vi "TPM with correction version 10-3-compare-1 scale factor_20180124.vi"() -> ()   [LabVIEW 2018]
uses:
  Casao LabVIEW SDK 1.0.5/Haso/Data Haso/Wavefront parameters.ctl
  Casao LabVIEW SDK 1.0.5/Casao/Casao/Loop prefs.ctl
  Casao LabVIEW SDK 1.0.5/Haso/Data Haso/DataHaso.ctl
  <vilib>/Utility/file.llb/Read From Spreadsheet File (DBL).vi
  <vilib>/Utility/file.llb/Write To Spreadsheet File (DBL).vi
panel:
  in  "Scale factor":dbl=1.0
  out "output path":path
  out "Model Coefficients (µm) after":sgl[](array[numeric])
  out "Model Coefficients (µm) before":sgl[](array[numeric])
  in  "stop":bool
  out "Slice now":dbl
  in  "Iteration #":u16(ring)=1 items=["1"=1, "2"=2, "3"=3, "4"=4, "5"=5]
  in  "AoExp Time":dbl(ring)=0.5 items=["0.2s"=0.2, "0.5s"=0.5, "1.0s"=1.0, "1.5s"=1.5]
  out "after correction":T1
  in  "Filter y tilt":bool=TRUE
  in  "Filter x tilt":bool=TRUE
  in  "Curvature filter":bool=TRUE
  out "PV":dbl
  out "RMS":dbl
  in  "Matrix path":path=path "F:/Min_Data/20180327_conf_calibration/CM32.aomc"
  in  "Offset path":path=path "F:/Min_Data/100nm bead correction.dat"
  out "Camera image":u32[][](graph)
  out "RMS":dbl
  out "PV":dbl
  out "before correction":T1
  in  "Curvature filter":bool=TRUE
  in  "Filter y tilt":bool=TRUE
  in  "Filter x tilt":bool=TRUE
  out "after correction":dbl[][](graph) caption="Wavefront"
  out "before correction":dbl[][](graph) caption="Wavefront"
  in  "ImExp Time (s)":dbl(ring)=0.5 items=["0.2"=0.2, "0.5"=0.5, "1.0"=1.0, "4.0"=4.0, "8.0"=8.0]
  in  "Step size(um)":dbl
  in  "Laser Power%(0-100)":dbl=50.0
  in  "Slices #":dbl=1.0
  in  "Average Frame #":dbl=10.0
  in  "Correction":bool
  # "OFF"
  # "ON"
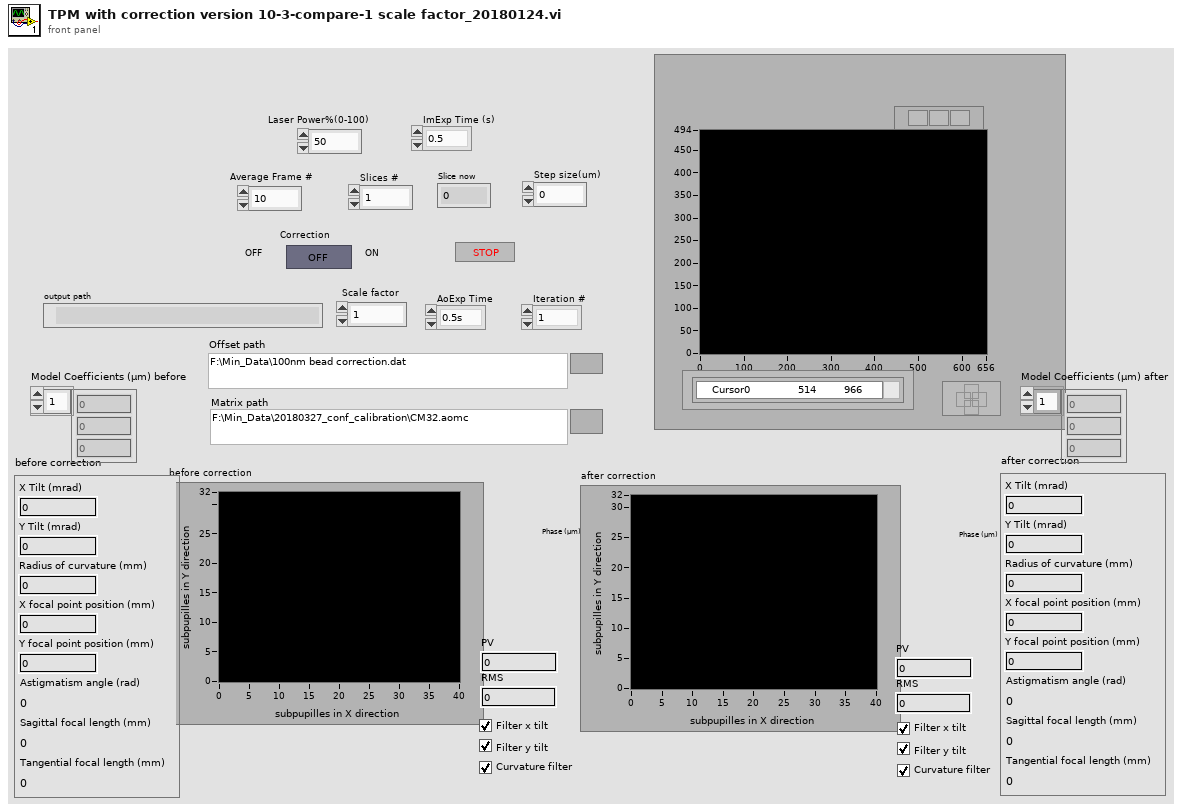
[diagram p1: front panel]
types:
  T1 = typedef "Wavefront parameters.ctl" = cluster{"X Tilt (mrad)":sgl, "Y Tilt (mrad)":sgl, "Radius of curvature (mm)":sgl, "X focal point position (mm)":sgl, "Y focal point position (mm)":sgl, "Astigmatism angle (rad)":sgl, "Sagittal focal length (mm)":sgl, "Tangential focal length (mm)":sgl}
  T2 = typedef "Loop prefs.ctl" = cluster{"Filter tilt on measurement (closed loop)":bool, "Correction gain (closed loop)":sgl, "Limit of subapertures off in CGP (%)":sgl, "Limit of saturated actuators (%)":sgl}
  T3 = cluster{"Filtre tilt X":bool, "Filtre tilt Y":bool, "Filtre courbure":bool}
  T4 = typedef "DataHaso.ctl" = i32
  T5 = cluster{"Measurement":T4, "Target":T4, "Manual target":T4}
  T6 = cluster{"Target for tilt":T4, "Target for focus":T4, "Target for all other aberrations":T4}
  T7 = typedef "Camera.ctl" = i32
  T8 = typedef "PhaseModul.ctl" = i32
  T9 = typedef "Haso.ctl" = i32
  T10 = typedef "Casao.ctl" = i32
  T11 = typedef "Image Compat.ctl" = cluster{"Signed/unsigned":bool, "Number of bits":T12, "Internal object id":i32, "Internal data id":i32}
  T12 = typedef "Data alignment enum.ctl" = enum16{"8", "16", "32"}
  T13 = typedef "Reconstruction prefs.ctl" = cluster{"Reconstruction type":enum16{"Modal", "Zonal"}, "Polynomial type":enum16{"Zernike", "Legendre"}, "Modal reconstruction prefs":T14, "Zonal reconstruction prefs":T17}
  T14 = typedef "Modal reconstruction prefs.ctl" = cluster{"Number of coefficients":u32, "Filtered coefficients":u32[], "RMS Zernike normalization":bool, "Matrix inversion method":u16, "Add zonal residual to modal fit ":bool, "Detection prefs":T15}
  T15 = typedef "PupilDetectionPrefs.ctl" = cluster{"Automatic pupil detection":bool, "Central occultation pupil":bool, "Semi-automatic pupil detection (find radius)":bool, "Semi-automatic pupil detection (find center)":bool, "Automatic pupil detection mode":enum16{"Contained", "Containing"}, "Start coordinates":cluster{"Pupil center (Zernike)":T16, "Pupil radius (Zernike)":sgl, "Pupil center (Legendre)":T16, "Pupil halfsize (Legendre)":T16}}
  T16 = typedef "Point2Df.ctl" = cluster{"X":sgl, "Y":sgl}
  T17 = typedef "Zonal reconstruction prefs.ctl" = cluster{"Number of weak iterations":u16, "Number of max iterations":u32, "Residual limit":sgl}
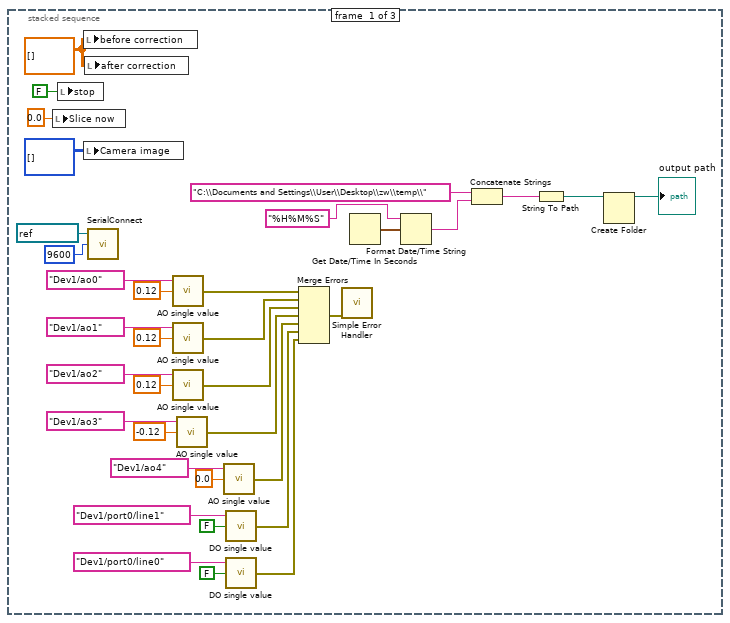
[diagram p2: hidden frame]
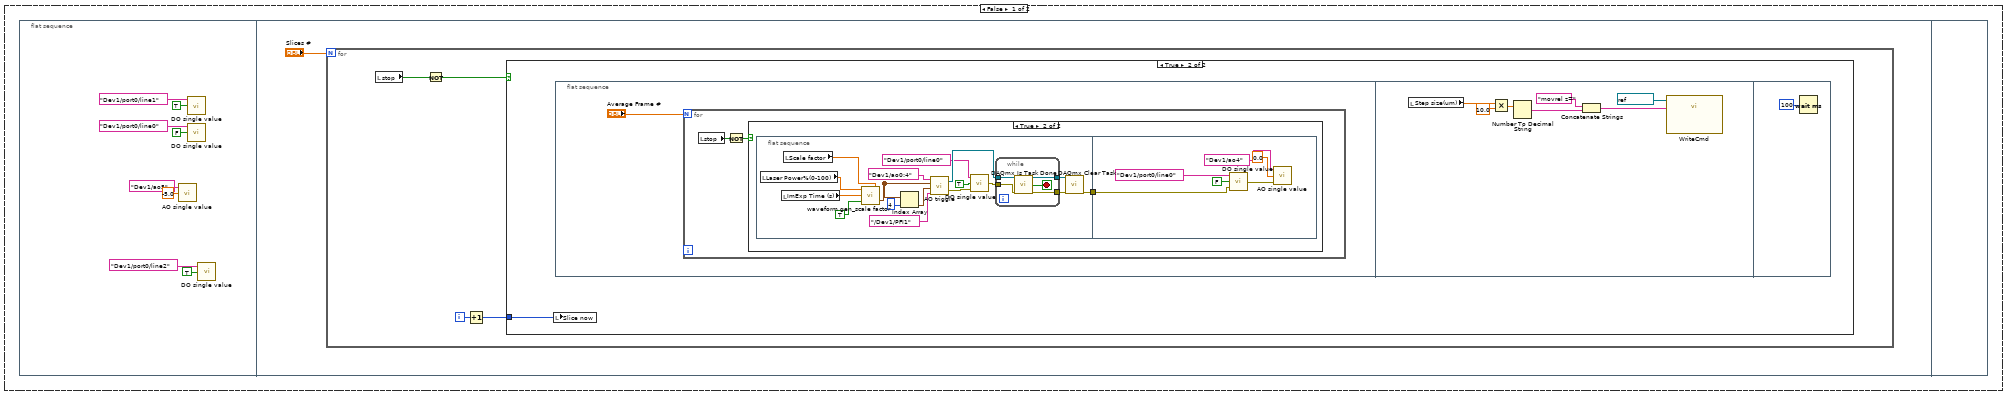
[diagram p3: hidden frame]
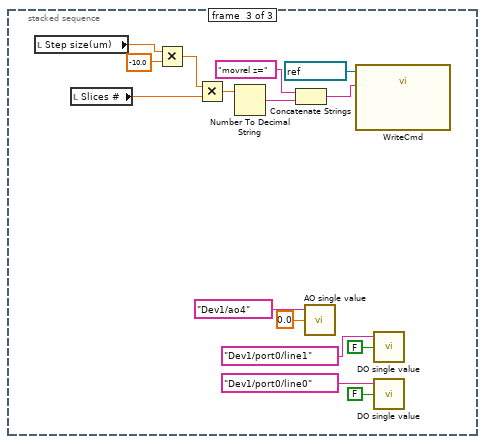
[diagram p11: hidden frame]
diagram:
  n1 = stacked-sequence {
    frame #0 {
      w34 = dbl[][] [] ("before correction")
      n2 = local write "Slice now"(0.0 ("Slice now")) -> ()
      n3 = local write "stop"(FALSE ("stop")) -> ()
      n4 = local write "before correction"(w34) -> ()
      n5 = local write "Camera image"(u32[][] [] ("Camera image")) -> ()
      n6 = local write "after correction"(w34) -> ()
      n7 = call "SerialConnect.vi"("baud rate (9600)"=u32 9600, "VISA resource name"=refnum<visa-resource-name> "COM1") -> ()  [unwired: 1 in, 3 out]
      n8 = call "AO single value.vi"("data"=0.12, "physical channels"=tag "Dev1/ao0") -> ("error out"=w17:errorcluster)  [unwired: 1 in]
      n9 = call "AO single value.vi"("data"=0.12, "physical channels"=tag "Dev1/ao1") -> ("error out"=w16:errorcluster)  [unwired: 1 in]
      n10 = call "AO single value.vi"("data"=0.12, "physical channels"=tag "Dev1/ao2") -> ("error out"=w15:errorcluster)  [unwired: 1 in]
      n11 = call "AO single value.vi"("data"=-0.12, "physical channels"=tag "Dev1/ao3") -> ("error out"=w14:errorcluster)  [unwired: 1 in]
      n12 = call "AO single value.vi"("data"=0.0, "physical channels"=tag "Dev1/ao4") -> ("error out"=w13:errorcluster)  [unwired: 1 in]
      n13 = call "DO single value.vi"("data"=FALSE, "lines"=tag "Dev1/port0/line1") -> ("error out"=w12:errorcluster)  [unwired: 1 in]
      n14 = call "DO single value.vi"("data"=FALSE, "lines"=tag "Dev1/port0/line0") -> ("error out"=w10:errorcluster)  [unwired: 1 in]
      n15 = Merge Errors(w17, w16, w15, w14, w13, w12, w10) -> (w11:errorcluster)
      n16 = call <vilib>:"Simple Error Handler.vi"("error in (no error)"=w11) -> ()  [unwired: 4 in, 5 out]
      n17 = Get Date/Time In Seconds() -> (seconds since 1Jan1904=w7:timestamp)
      n18 = Format Date/Time String(time format string (%c)="%H%M%S", seconds (now)=w7) -> (date/time string=w4:string)  [unwired: 1 in]
      n19 = Concatenate Strings("C:\\Documents and Settings\\User\\Desktop\\zw\\temp\\" ("string"), w4) -> (w3:string)
      n20 = String To Path(string=w3) -> (path=w2:path)
      n21 = Create Folder(path (use dialog)=w2) -> (created path=→"output path":path)  [unwired: 2 in, 2 out]
    }
    frame #1 {
      n22 = case shown="True" "Correction" {
        frame False {
          n23 = flat-sequence {
            frame #0 {
              n24 = call "AO single value.vi"("data"=-5.0, "physical channels"=tag "Dev1/ao5") -> ()  [unwired: 1 in, 1 out]
              n25 = call "DO single value.vi"("data"=TRUE, "lines"=tag "Dev1/port0/line1") -> ()  [unwired: 1 in, 1 out]
              n26 = call "DO single value.vi"("data"=FALSE, "lines"=tag "Dev1/port0/line0") -> ()  [unwired: 1 in, 1 out]
              n27 = call "DO single value.vi"("data"=TRUE, "lines"=tag "Dev1/port0/line2") -> ()  [unwired: 1 in, 1 out]
            }
            frame #1 {
              n28 = for {
                N: "Slices #" -> [_]
                i -> [w49]
                n29 = local read "stop"() -> (w47:bool)
                n30 = Not(x=w47) -> (.not. x?=w46:bool)
                n31 = Increment(x=w49) -> (x+1=w48:i32)
                n32 = case shown="True" w46 {
                  tunnel: w48 -> [_ w50]
                  frame False {
                  }
                  frame True {
                    n33 = local write "Slice now"(w50) -> ()
                    n34 = flat-sequence {
                      frame #0 {
                        n35 = for {
                          N: "Average Frame #" -> [_]
                          n36 = local read "stop"() -> (w52:bool)
                          n37 = Not(x=w52) -> (.not. x?=w53:bool)
                          n38 = case shown="True" w53 {
                            frame False {
                            }
                            frame True {
                              n39 = flat-sequence {
                                tunnel: [w60] -> w54
                                tunnel: w54 -> [w78]
                                frame #0 {
                                n40 = local read "Laser Power%(0-100)"() -> (w56:dbl)
                                n41 = local read "ImExp Time (s)"() -> (w57:dbl)
                                n42 = local read "Scale factor"() -> (w55:dbl)
                                n43 = call "waveform gen_scale factor.vi"("Scale factor"=w55, "Boolean"=TRUE, "Exposure Time (s)"=w57, "Laser Power%(0-100)"=w56) -> ("waveform"=w59:waveform(dbl)[])
                                n44 = Index Array(array=w59, index=4) -> (element=w68:waveform(dbl))
                                n45 = call "AO triggle.vi"("physical channels"=tag "Dev1/ao0:4", "data"=w59, "waveform"=w68, "trig source"=tag "/Dev1/PFI1") -> ("task out"=w65:refnum<k21>, "error out"=w62:errorcluster)  [unwired: 1 in]
                                n46 = call "DO single value.vi"("error in"=w62, "data"=TRUE, "lines"=tag "Dev1/port0/line0") -> ("error out"=w61:errorcluster)
                                n47 = while {
                                tunnel: [w76] -> w71
                                tunnel: [w75] -> w70
                                tunnel: w65 -> [w73]
                                tunnel: w61 -> [w72]
                                stop <- w74 stop-if-true
                                n48 = call <vilib>:"DAQmx Is Task Done.vi"("task/channels in"=w73, "error in"=w72) -> ("task out"=w76:refnum<k21>, "task done?"=w74:bool, "error out"=w75:errorcluster)  [unwired: 11 in]
                                }
                                n49 = call <vilib>:"DAQmx Clear Task.vi"("task in"=w71, "error in"=w70) -> ("error out"=w60:errorcluster)  [unwired: 13 in]
                                }
                                frame #1 {
                                n50 = call "DO single value.vi"("error in"=w78, "data"=FALSE, "lines"=tag "Dev1/port0/line0") -> ("error out"=w77:errorcluster)
                                n51 = call "AO single value.vi"("error in"=w77, "data"=0.0, "physical channels"=tag "Dev1/ao4") -> ()  [unwired: 1 out]
                                }
                              }
                            }
                          }
                        }
                      }
                      frame #1 {
                        n52 = local read "Step size(um)"() -> (w83:dbl)
                        n53 = Multiply(x=w83, y=10.0) -> (x*y=w85:dbl)
                        n54 = Number To Decimal String(number=w85) -> (decimal integer string=w88:string)  [unwired: 1 in]
                        n55 = Concatenate Strings("movrel z=", w88) -> (w87:string)
                        n56 = call "WriteCmd.vi"("Command"=w87, "VISA resource name"=refnum<visa-resource-name> "COM1") -> ()  [unwired: 1 in, 1 out]
                      }
                      frame #2 {
                        n57 = Wait (ms)(milliseconds to wait=u32 100) -> ()  [unwired: 1 out]
                      }
                    }
                  }
                }
              }
            }
            frame #2 {
            }
          }
        }
        frame True {
          n58 = flat-sequence {
            tunnel: [w106] -> w98
            tunnel: [w108] -> w97
            tunnel: [w107] -> w96
            tunnel: [w106] -> w95
            tunnel: [w105] -> w94
            tunnel: [w104] -> w92
            tunnel: [w99] -> w91
            tunnel: w98 -> [w125]
            tunnel: w97 -> [w124]
            tunnel: w96 -> [w123]
            tunnel: w95 -> [w119]
            tunnel: w94 -> [w117]
            tunnel: [w122] -> w93
            tunnel: w92 -> [w121]
            tunnel: w91 -> [w115]
            tunnel: w93 -> [w651]
            frame #0 {
              n59 = call "AO single value.vi"("data"=0.0, "physical channels"=tag "Dev1/ao4") -> ()  [unwired: 1 in, 1 out]
              n60 = local read "AoExp Time"() -> (w109:dbl)
              n61 = call-poly <vilib>:"Read From Spreadsheet File.vi"("format (%.3f)"="%.8f", "file path (dialog if empty)"="Offset path") -> ("first row"=w99:dbl[])  [unwired: 5 in, 4 out]
              n62 = call "DO single value.vi"("data"=TRUE, "lines"=tag "Dev1/port0/line1") -> ()  [unwired: 1 in, 1 out]
              n63 = call "DO single value.vi"("data"=FALSE, "lines"=tag "Dev1/port0/line0") -> ()  [unwired: 1 in, 1 out]
              n64 = call "AO init.vi"("Exposure duration specified (s)"=w109, "Commands in"=w99, "Matrix path"="Matrix path") -> ("error out"=w106:errorcluster, "Camera"=w108:T7, "Mirror"=w104:T8, "Haso"=w107:T9, "Casao"=w105:T10)  [unwired: 3 in, 1 out]
            }
            frame #1 {
              n65 = local read "Slices #"() -> (w126:dbl)
              n66 = call "Casao Set Preferences.vi"("error in (no error)"=w119, "Loop preferences"=T2 {"Filter tilt on measurement (closed loop)"=FALSE, "Correction gain (closed loop)"=0.75, "Limit of subapertures off in CGP (%)"=0.0, "Limit of saturated actuators (%)"=0.0}, "Casao"=w117) -> ("error out"=w118:errorcluster, "Casao (dup)"=w116:T10)  [unwired: 3 in]
              n67 = for {
                N: w126 -> [_]
                tunnel: w125 -> [w142]
                tunnel: w124 -> [w141]
                tunnel: w123 -> [w140]
                tunnel: w118 -> [w128]
                tunnel: [w139] -> w122
                tunnel: w121 -> [w130]
                tunnel: w116 -> [w138]
                tunnel: w115 -> [w131]
                i -> [w134]
                n68 = local read "stop"() -> (w136:bool)
                n69 = call "PhaseModul apply command.vi"("error in (no error)"=w128, "Commands in"=w131, "Mirror"=w130) -> ("error out"=w127:errorcluster, "Mirror (dup)"=w129:T8)  [unwired: 2 in, 1 out]
                n70 = Increment(x=w134) -> (x+1=w137:i32)
                n71 = local write "Slice now"(w137) -> ()
                n72 = Not(x=w136) -> (.not. x?=w135:bool)
                n73 = case shown="True" w135 {
                  tunnel: w142 -> [_ w177]
                  tunnel: w141 -> [_ w176]
                  tunnel: w140 -> [_ w175]
                  tunnel: w127 -> [_ w174]
                  tunnel: [w143 w171] -> w139
                  tunnel: w129 -> [_ w173]
                  tunnel: w138 -> [w143 w172]
                  frame False {
                  }
                  frame True {
                    n74 = flat-sequence {
                      tunnel: w172 -> [w182]
                      tunnel: w173 -> [w183]
                      tunnel: w174 -> [w184]
                      tunnel: w175 -> [w185]
                      tunnel: w176 -> [w186]
                      tunnel: w177 -> [w187]
                      tunnel: [w187] -> w149
                      tunnel: [w186] -> w148
                      tunnel: [w185] -> w147
                      tunnel: [w184] -> w146
                      tunnel: [w183] -> w145
                      tunnel: [w182] -> w144
                      tunnel: [w222] -> w170
                      tunnel: [w221] -> w169
                      tunnel: [w220] -> w168
                      tunnel: [w215] -> w167
                      tunnel: [w216] -> w166
                      tunnel: [w217] -> w165
                      tunnel: w149 -> [w222]
                      tunnel: w148 -> [w221]
                      tunnel: w147 -> [w220]
                      tunnel: w146 -> [w216]
                      tunnel: w145 -> [w217]
                      tunnel: w144 -> [w215]
                      tunnel: w170 -> [w264]
                      tunnel: w169 -> [w263]
                      tunnel: w168 -> [w262]
                      tunnel: w167 -> [w261]
                      tunnel: w166 -> [w260]
                      tunnel: [w240] -> w164
                      tunnel: [w239] -> w163
                      tunnel: [w235] -> w162
                      tunnel: [w233] -> w161
                      tunnel: [w231] -> w160
                      tunnel: w165 -> [w226]
                      tunnel: [w225] -> w159
                      tunnel: [w223] -> w158
                      tunnel: w164 -> [w406]
                      tunnel: w163 -> [w405]
                      tunnel: w162 -> [w403]
                      tunnel: w161 -> [w402]
                      tunnel: w160 -> [w401]
                      tunnel: [w400] -> w157
                      tunnel: w159 -> [w399]
                      tunnel: [w398] -> w156
                      tunnel: [w397] -> w155
                      tunnel: [w396] -> w154
                      tunnel: [w395] -> w153
                      tunnel: [w394] -> w152
                      tunnel: w158 -> [w393]
                      tunnel: [w393] -> w151
                      tunnel: w157 -> [w613]
                      tunnel: [w613] -> w150
                      tunnel: w156 -> [w603]
                      tunnel: w155 -> [w602]
                      tunnel: w154 -> [w601]
                      tunnel: w153 -> [w591]
                      tunnel: w152 -> [w592]
                      tunnel: w151 -> [w590]
                      tunnel: w150 -> [w614]
                      tunnel: [w614] -> w171
                      frame #0 {
                        n75 = local read "Average Frame #"() -> (w181:dbl)
                        n76 = Wait (ms)(milliseconds to wait=u32 100) -> ()  [unwired: 1 out]
                        n77 = call "AO single value.vi"("data"=-5.0, "physical channels"=tag "Dev1/ao5") -> ()  [unwired: 1 in, 1 out]
                        n78 = for {
                          N: w181 -> [_]
                          n79 = local read "stop"() -> (w188:bool)
                          n80 = Not(x=w188) -> (.not. x?=w189:bool)
                          n81 = case shown="True" w189 {
                            frame False {
                            }
                            frame True {
                              n82 = flat-sequence {
                                frame #0 {
                                n83 = local read "Laser Power%(0-100)"() -> (w191:dbl)
                                n84 = local read "ImExp Time (s)"() -> (w192:dbl)
                                n85 = local read "Scale factor"() -> (w190:dbl)
                                n86 = call "waveform gen_scale factor.vi"("Scale factor"=w190, "Boolean"=TRUE, "Exposure Time (s)"=w192, "Laser Power%(0-100)"=w191) -> ("waveform"=w194:waveform(dbl)[])
                                n87 = Index Array(array=w194, index=4) -> (element=w202:waveform(dbl))
                                n88 = call "AO triggle.vi"("physical channels"=tag "Dev1/ao0:4", "data"=w194, "waveform"=w202, "trig source"=tag "/Dev1/PFI1") -> ("task out"=w199:refnum<k21>, "error out"=w196:errorcluster)  [unwired: 1 in]
                                n89 = call "DO single value.vi"("error in"=w196, "data"=TRUE, "lines"=tag "Dev1/port0/line0") -> ("error out"=w195:errorcluster)
                                n90 = while {
                                tunnel: [w210] -> w205
                                tunnel: [w209] -> w204
                                tunnel: w199 -> [w207]
                                tunnel: w195 -> [w206]
                                stop <- w208 stop-if-true
                                n91 = call <vilib>:"DAQmx Is Task Done.vi"("task/channels in"=w207, "error in"=w206) -> ("task out"=w210:refnum<k21>, "task done?"=w208:bool, "error out"=w209:errorcluster)  [unwired: 11 in]
                                }
                                n92 = call <vilib>:"DAQmx Clear Task.vi"("task in"=w205, "error in"=w204) -> ()  [unwired: 13 in, 1 out]
                                }
                                frame #1 {
                                n93 = call "AO single value.vi"("data"=0.0, "physical channels"=tag "Dev1/ao4") -> ()  [unwired: 1 in, 1 out]
                                n94 = call "DO single value.vi"("data"=FALSE, "lines"=tag "Dev1/port0/line0") -> ()  [unwired: 1 in, 1 out]
                                }
                              }
                            }
                          }
                        }
                      }
                      frame #1 {
                        n95 = call "AO single value.vi"("data"=1.0, "physical channels"=tag "Dev1/ao5") -> ()  [unwired: 1 in, 1 out]
                      }
                      frame #2 {
                        n96 = flat-sequence {
                          tunnel: [w273] -> w259
                          tunnel: [w272] -> w258
                          tunnel: [w271] -> w257
                          tunnel: [w270] -> w256
                          tunnel: [w269] -> w255
                          tunnel: w262 -> [w271]
                          tunnel: w263 -> [w272]
                          tunnel: w264 -> [w273]
                          tunnel: [w268] -> w254
                          tunnel: w261 -> [w268]
                          tunnel: [w267] -> w253
                          tunnel: w260 -> [w267]
                          tunnel: [w266] -> w227
                          tunnel: w226 -> [w266]
                          tunnel: w259 -> [w289]
                          tunnel: w258 -> [w290]
                          tunnel: w257 -> [w291]
                          tunnel: [w291] -> w252
                          tunnel: [w288] -> w251
                          tunnel: [w287] -> w250
                          tunnel: [w286] -> w249
                          tunnel: w256 -> [w286]
                          tunnel: [w285] -> w248
                          tunnel: w255 -> [w285]
                          tunnel: [w284] -> w247
                          tunnel: w254 -> [w284]
                          tunnel: [w283] -> w246
                          tunnel: w253 -> [w283]
                          tunnel: [w282] -> w228
                          tunnel: w227 -> [w282]
                          tunnel: w252 -> [w303]
                          tunnel: [w303] -> w243
                          tunnel: [w302] -> w244
                          tunnel: w251 -> [w302]
                          tunnel: [w301] -> w245
                          tunnel: w250 -> [w301]
                          tunnel: w249 -> [w296]
                          tunnel: w248 -> [w295]
                          tunnel: [w294] -> w242
                          tunnel: w247 -> [w294]
                          tunnel: [w293] -> w241
                          tunnel: w246 -> [w293]
                          tunnel: [w292] -> w229
                          tunnel: w228 -> [w292]
                          tunnel: w245 -> [w385]
                          tunnel: w244 -> [w345]
                          tunnel: w243 -> [w346]
                          tunnel: w242 -> [w371]
                          tunnel: w241 -> [w370]
                          tunnel: [w349] -> w238
                          tunnel: [w348] -> w237
                          tunnel: [w347] -> w236
                          tunnel: [w346] -> w234
                          tunnel: [w345] -> w232
                          tunnel: [w344] -> w230
                          tunnel: w229 -> [w343]
                          tunnel: [w343] -> w224
                          tunnel: [w317] -> w223
                          tunnel: [w391] -> w239
                          tunnel: [w392] -> w240
                          tunnel: w238 -> [w392]
                          tunnel: w237 -> [w391]
                          tunnel: w236 -> [w390]
                          tunnel: [w389] -> w235
                          tunnel: w234 -> [w389]
                          tunnel: [w388] -> w233
                          tunnel: w232 -> [w388]
                          tunnel: [w387] -> w231
                          tunnel: w230 -> [w387]
                          tunnel: [w386] -> w225
                          tunnel: w224 -> [w386]
                          frame #0 {
                            n97 = local read "Laser Power%(0-100)"() -> (w279:dbl)
                            n98 = local read "AoExp Time"() -> (w278:dbl)
                            n99 = local read "Scale factor"() -> (w265:dbl)
                            n100 = call "waveform gen_scale factor.vi"("Scale factor"=w265, "Boolean"=FALSE, "Exposure Time (s)"=w278, "Laser Power%(0-100)"=w279) -> ("waveform"=w277:waveform(dbl)[])
                            n101 = Index Array(array=w277, index=4) -> (element=w276:waveform(dbl))
                            n102 = call "AO triggle.vi"("physical channels"=tag "Dev1/ao0:4", "data"=w277, "waveform"=w276, "trig source"=tag "/Dev1/PFI1") -> ("task out"=w270:refnum<k21>, "error out"=w269:errorcluster)  [unwired: 1 in]
                          }
                          frame #1 {
                            n103 = call "Camera Start.vi"("error in (no error)"=w289, "camera"=w290) -> ("error out"=w287:errorcluster, "camera (dup)"=w288:T7)  [unwired: 4 in]
                          }
                          frame #2 {
                            n104 = while {
                              tunnel: [w308] -> w298
                              tunnel: [w307] -> w297
                              tunnel: w296 -> [w305]
                              tunnel: w295 -> [w304]
                              stop <- w306 stop-if-true
                              n105 = call <vilib>:"DAQmx Is Task Done.vi"("task/channels in"=w305, "error in"=w304) -> ("task out"=w308:refnum<k21>, "task done?"=w306:bool, "error out"=w307:errorcluster)  [unwired: 11 in]
                            }
                            n106 = call "DO single value.vi"("data"=TRUE, "lines"=tag "Dev1/port0/line0") -> ()  [unwired: 1 in, 1 out]
                            n107 = call <vilib>:"DAQmx Clear Task.vi"("task in"=w298, "error in"=w297) -> ()  [unwired: 13 in, 1 out]
                          }
                          frame #3 {
                            n108 = call "Camera Get image.vi"("error in (no error)"=w385, "camera"=w345) -> ("error out"=w367:errorcluster, "Image"=w368:T11, "camera (dup)"=w369:T7)  [unwired: 3 in]
                            n109 = call "Camera Stop.vi"("error in (no error)"=w367, "camera"=w369) -> ()  [unwired: 4 in, 2 out]
                            n110 = call "Image get data.vi"("error in (no error)"=w367, "Image Compat"=w368) -> ("error out"=w357:errorcluster, "Array"=w366:u32[][], "Image Compat (dup)"=w356:T11)  [unwired: 3 in]
                            n111 = call "AO single value.vi"("data"=0.0, "physical channels"=tag "Dev1/ao4") -> ()  [unwired: 1 in, 1 out]
                            n112 = local write "Camera image"(w366) -> ()
                            n113 = call "Haso compute slopes.vi"("error in (no error)"=w357, "Image Compat"=w356, "Haso"=w346) -> ("error out"=w315:errorcluster, "Data Haso"=w319:T4)  [unwired: 1 in, 2 out]
                            n114 = call "DO single value.vi"("data"=FALSE, "lines"=tag "Dev1/port0/line0") -> ()  [unwired: 1 in, 1 out]
                            n115 = call "DataHaso ctor copie.vi"("error in (no error)"=w315, "DataHaso"=w319) -> ("error out"=w314:errorcluster, "new DataHaso"=w317:T4, "DataHaso (dup)"=w316:T4)  [unwired: 3 in]
                            n116 = call "DataHaso get reconstruction prefs.vi"("error in (no error)"=w314, "Data Haso"=w316) -> ("error out"=w330:errorcluster, "Reconstruction Preferences"=w326:T13, "Data Haso (dup)"=w329:T4)  [unwired: 3 in]
                            n117 = Bundle By Name(cluster=w326, "Reconstruction type"=enum16{"Modal", "Zonal"}."Modal", "Polynomial type"=enum16{"Zernike", "Legendre"}."Zernike", "Modal reconstruction prefs.Number of coefficients"=u32 32) -> (w325:T13)
                            n118 = call "DataHaso set reconstruction prefs.vi"("error in (no error)"=w330, "Reconstruction Preferences"=w325, "Data Haso"=w329) -> ("error out"=w327:errorcluster, "Data Haso (dup)"=w328:T4)  [unwired: 3 in]
                            n119 = call "DataHaso get modal coefficients.vi"("error in (no error)"=w327, "Data Haso"=w328) -> ("error out"=w320:errorcluster, "Coefficients (µm)"=w331:sgl[], "Data Haso (dup)"=w321:T4)  [unwired: 3 in]
                            "Model Coefficients (µm) before" <- w331
                            n120 = Bundle By Name(cluster=T3 {"Filtre tilt X"=FALSE, "Filtre tilt Y"=FALSE, "Filtre courbure"=FALSE} ("Filtre"), "Filtre tilt X"="Filter x tilt", "Filtre tilt Y"="Filter y tilt", "Filtre courbure"="Curvature filter") -> (w351:T3)
                            n121 = call "DataHaso parameters.vi"("error in (no error)"=w320, "Data Haso"=w321) -> ("error out"=w364:errorcluster, "Parameters"=w339:T1, "Data Haso (dup)"=w365:T4)  [unwired: 3 in]
                            "before correction" <- w339
                            n122 = control-ref of="before correction"() -> (w350:refnum<vi>)
                            n123 = Cluster To Array(cluster=w339) -> (array=w340:sgl[])
                            n124 = call "DataHaso filter tilt or curvature.vi"("error in (no error)"=w364, "Filter (default: all true)"=w351, "Data Haso"=w365) -> ("error out"=w362:errorcluster, "Data Haso (dup)"=w363:T4)  [unwired: 3 in]
                            n125 = local read "Slice now"() -> (w333:dbl)
                            n126 = call "DataHaso phase.vi"("error in (no error)"=w362, "Data Haso"=w363) -> ("error out"=w360:errorcluster, "Phase (µm)"=w361:i32, "Data Haso (dup)"=w318:T4)  [unwired: 3 in]
                            n127 = Number To Decimal String(number=w333) -> (decimal integer string=w335:string)  [unwired: 1 in]
                            n128 = call "Formatter Intensity Graph.vi"("error in (no error)"=w360, "Intensity Graph"=w350, "Surface with pupil"=w361) -> ("error out"=w358:errorcluster, "Surface with pupil (dup)"=w359:i32)  [unwired: 2 in, 1 out]
                            n129 = call "Surface with pupil get stats.vi"("error in (no error)"=w358, "Surface Avec Pupille"=w359) -> ("error out"=w344:errorcluster, "PV"=w342:sgl, "RMS"=w341:dbl)  [unwired: 2 in, 1 out]
                            "PV" <- w342
                            "RMS" <- w341
                            n130 = local read "output path"() -> (w311:path)
                            n131 = Concatenate Strings("before_slice", w335, ".dat") -> (w310:string)
                            n132 = Build Path(base path=w311, name or relative path=w310) -> (appended path=w309:path)
                            n133 = Build Array (concatenate)(w342, w341, w340, w331) -> (w338:dbl[])
                            n134 = Merge Errors(w344, w370) -> (w380:errorcluster)
                            n135 = Bundle By Name(cluster=T6 {"Target for tilt"=0, "Target for focus"=0, "Target for all other aberrations"=0} ("References"), "Target for tilt"=w317, "Target for focus"=w317) -> (w383:T6)
                            n136 = call "DataHaso ctor copie.vi"("error in (no error)"=w380, "DataHaso"=w318) -> ("error out"=w382:errorcluster, "new DataHaso"=w381:T4)  [unwired: 3 in, 1 out]
                            n137 = call-poly <vilib>:"Write To Spreadsheet File.vi"("transpose? (no:F)"=TRUE, "format (%.3f)"="%.6f", "1D data"=w338, "file path (dialog if empty)"=w309) -> ()  [unwired: 4 in, 1 out]
                            n138 = call "Casao Compute target.vi"("error in (no error)"=w382, "Targets"=w383, "DataHaso"=w381, "Casao"=w371) -> ("error out"=w378:errorcluster, "DataHaso (dup)"=w347:T4, "Casao (dup)"=w379:T10)  [unwired: 1 out]
                            n139 = Bundle By Name(cluster=T5 {"Measurement"=0, "Target"=0, "Manual target"=0} ("Slopes"), "Measurement"=w318, "Target"=w347) -> (w377:T5)
                            n140 = call "Casao get correction commands.vi"("Casao"=w379, "Slopes"=w377, "error in (no error)"=w378) -> ("Casao (dup)"=w349:T10, "Commands"=w374:sgl[], "error out"=w375:errorcluster)  [unwired: 2 in, 2 out]
                            n141 = call "PhaseModul apply command.vi"("error in (no error)"=w375, "Commands in"=w374, "Mirror"=w343) -> ("error out"=w348:errorcluster)  [unwired: 2 in, 2 out]
                          }
                          frame #4 {
                            n142 = call "DataHaso dtor.vi"("Data Haso"=w390) -> ()  [unwired: 6 in, 1 out]
                          }
                        }
                      }
                      frame #3 {
                        n143 = for {
                          N: "Iteration #" -> [_]
                          tunnel: w406 -> [w435]
                          tunnel: w405 -> [w434]
                          tunnel: w403 -> [w433]
                          tunnel: w402 -> [w432]
                          tunnel: w401 -> [w431]
                          tunnel: [w429] -> w400
                          tunnel: w399 -> [w424]
                          tunnel: [w423] -> w398
                          tunnel: [w421] -> w397
                          tunnel: [w419] -> w396
                          tunnel: [w417] -> w395
                          tunnel: [w414] -> w394
                          tunnel: w393 -> [w413]
                          i -> [w412]
                          n144 = Increment(x=w412) -> (x+1=w411:i32)
                          n145 = flat-sequence {
                            tunnel: [w460] -> w454
                            tunnel: [w461] -> w453
                            tunnel: [w462] -> w452
                            tunnel: [w466] -> w451
                            tunnel: [w465] -> w450
                            tunnel: [w464] -> w449
                            tunnel: [w463] -> w448
                            tunnel: w435 -> [w464]
                            tunnel: w434 -> [w463]
                            tunnel: w433 -> [w462]
                            tunnel: w432 -> [w461]
                            tunnel: w431 -> [w460]
                            tunnel: [w459] -> w425
                            tunnel: w424 -> [w459]
                            tunnel: w411 -> [w457]
                            tunnel: [w456] -> w408
                            tunnel: w454 -> [w483]
                            tunnel: w453 -> [w484]
                            tunnel: w452 -> [w485]
                            tunnel: [w485] -> w447
                            tunnel: [w482] -> w446
                            tunnel: [w481] -> w445
                            tunnel: [w480] -> w444
                            tunnel: w451 -> [w480]
                            tunnel: [w479] -> w443
                            tunnel: w450 -> [w479]
                            tunnel: [w478] -> w442
                            tunnel: w449 -> [w478]
                            tunnel: [w477] -> w441
                            tunnel: w448 -> [w477]
                            tunnel: [w476] -> w426
                            tunnel: w425 -> [w476]
                            tunnel: [w475] -> w409
                            tunnel: w408 -> [w475]
                            tunnel: w447 -> [w498]
                            tunnel: [w498] -> w438
                            tunnel: [w497] -> w439
                            tunnel: w446 -> [w497]
                            tunnel: [w496] -> w440
                            tunnel: w445 -> [w496]
                            tunnel: w444 -> [w491]
                            tunnel: w443 -> [w490]
                            tunnel: [w489] -> w437
                            tunnel: w442 -> [w489]
                            tunnel: [w488] -> w436
                            tunnel: w441 -> [w488]
                            tunnel: [w487] -> w427
                            tunnel: w426 -> [w487]
                            tunnel: [w486] -> w410
                            tunnel: w409 -> [w486]
                            tunnel: w440 -> [w566]
                            tunnel: w439 -> [w567]
                            tunnel: w438 -> [w568]
                            tunnel: w437 -> [w553]
                            tunnel: w436 -> [w552]
                            tunnel: [w532] -> w430
                            tunnel: [w531] -> w428
                            tunnel: w427 -> [w511]
                            tunnel: [w527] -> w422
                            tunnel: [w526] -> w420
                            tunnel: [w525] -> w418
                            tunnel: [w524] -> w416
                            tunnel: [w513] -> w415
                            tunnel: w413 -> [w510]
                            tunnel: w410 -> [w507]
                            tunnel: [w504] -> w407
                            tunnel: w430 -> [w580]
                            tunnel: [w579] -> w429
                            tunnel: w428 -> [w579]
                            tunnel: [w578] -> w423
                            tunnel: w422 -> [w578]
                            tunnel: [w577] -> w421
                            tunnel: w420 -> [w577]
                            tunnel: [w576] -> w419
                            tunnel: w418 -> [w576]
                            tunnel: [w572] -> w417
                            tunnel: w416 -> [w573]
                            tunnel: w415 -> [w575]
                            tunnel: [w575] -> w414
                            tunnel: w407 -> [w574]
                            frame #0 {
                              n146 = local read "Laser Power%(0-100)"() -> (w472:dbl)
                              n147 = local read "AoExp Time"() -> (w471:dbl)
                              n148 = local read "Scale factor"() -> (w455:dbl)
                              n149 = call "waveform gen_scale factor.vi"("Scale factor"=w455, "Boolean"=FALSE, "Exposure Time (s)"=w471, "Laser Power%(0-100)"=w472) -> ("waveform"=w470:waveform(dbl)[])
                              n150 = local read "Iteration #"() -> (w458:u16)
                              n151 = Index Array(array=w470, index=4) -> (element=w469:waveform(dbl))
                              n152 = Less?(x=w458, y=w457) -> (x < y?=w456:bool)
                              n153 = call "AO triggle.vi"("physical channels"=tag "Dev1/ao0:4", "data"=w470, "waveform"=w469, "trig source"=tag "/Dev1/PFI1") -> ("task out"=w466:refnum<k21>, "error out"=w465:errorcluster)  [unwired: 1 in]
                            }
                            frame #1 {
                              n154 = call "Camera Start.vi"("error in (no error)"=w483, "camera"=w484) -> ("error out"=w481:errorcluster, "camera (dup)"=w482:T7)  [unwired: 4 in]
                            }
                            frame #2 {
                              n155 = while {
                                tunnel: [w503] -> w493
                                tunnel: [w502] -> w492
                                tunnel: w491 -> [w500]
                                tunnel: w490 -> [w499]
                                stop <- w501 stop-if-true
                                n156 = call <vilib>:"DAQmx Is Task Done.vi"("task/channels in"=w500, "error in"=w499) -> ("task out"=w503:refnum<k21>, "task done?"=w501:bool, "error out"=w502:errorcluster)  [unwired: 11 in]
                              }
                              n157 = call "DO single value.vi"("data"=TRUE, "lines"=tag "Dev1/port0/line0") -> ()  [unwired: 1 in, 1 out]
                              n158 = call <vilib>:"DAQmx Clear Task.vi"("task in"=w493, "error in"=w492) -> ()  [unwired: 13 in, 1 out]
                            }
                            frame #3 {
                              n159 = call "Camera Get image.vi"("error in (no error)"=w566, "camera"=w567) -> ("error out"=w549:errorcluster, "Image"=w550:T11, "camera (dup)"=w551:T7)  [unwired: 3 in]
                              n160 = call "Camera Stop.vi"("error in (no error)"=w549, "camera"=w551) -> ()  [unwired: 4 in, 2 out]
                              n161 = call "Image get data.vi"("error in (no error)"=w549, "Image Compat"=w550) -> ("error out"=w539:errorcluster, "Array"=w548:u32[][], "Image Compat (dup)"=w538:T11)  [unwired: 3 in]
                              n162 = call "AO single value.vi"("data"=0.0, "physical channels"=tag "Dev1/ao4") -> ()  [unwired: 1 in, 1 out]
                              n163 = local write "Camera image"(w548) -> ()
                              n164 = call "Haso compute slopes.vi"("error in (no error)"=w539, "Image Compat"=w538, "Haso"=w568) -> ("error out"=w516:errorcluster, "Data Haso"=w515:T4)  [unwired: 1 in, 2 out]
                              n165 = call "DO single value.vi"("data"=FALSE, "lines"=tag "Dev1/port0/line0") -> ()  [unwired: 1 in, 1 out]
                              n166 = call "DataHaso get reconstruction prefs.vi"("error in (no error)"=w516, "Data Haso"=w515) -> ("error out"=w522:errorcluster, "Reconstruction Preferences"=w521:T13, "Data Haso (dup)"=w523:T4)  [unwired: 3 in]
                              n167 = Bundle By Name(cluster=w521, "Reconstruction type"=enum16{"Modal", "Zonal"}."Modal", "Polynomial type"=enum16{"Zernike", "Legendre"}."Zernike", "Modal reconstruction prefs.Number of coefficients"=u32 32) -> (w520:T13)
                              n168 = call "DataHaso set reconstruction prefs.vi"("error in (no error)"=w522, "Reconstruction Preferences"=w520, "Data Haso"=w523) -> ("error out"=w508:errorcluster, "Data Haso (dup)"=w509:T4)  [unwired: 3 in]
                              n169 = call "DataHaso get modal coefficients.vi"("error in (no error)"=w508, "Data Haso"=w509) -> ("error out"=w514:errorcluster, "Coefficients (µm)"=w513:sgl[], "Data Haso (dup)"=w512:T4)  [unwired: 3 in]
                              "Model Coefficients (µm) after" <- w513
                              n170 = Bundle By Name(cluster=T3 {"Filtre tilt X"=FALSE, "Filtre tilt Y"=FALSE, "Filtre courbure"=FALSE} ("Filtre"), "Filtre tilt X"="Filter x tilt", "Filtre tilt Y"="Filter y tilt", "Filtre courbure"="Curvature filter") -> (w536:T3)
                              n171 = call "DataHaso parameters.vi"("error in (no error)"=w514, "Data Haso"=w512) -> ("error out"=w546:errorcluster, "Parameters"=w525:T1, "Data Haso (dup)"=w547:T4)  [unwired: 3 in]
                              "after correction" <- w525
                              n172 = control-ref of="after correction"() -> (w530:refnum<vi>)
                              n173 = call "DataHaso filter tilt or curvature.vi"("error in (no error)"=w546, "Filter (default: all true)"=w536, "Data Haso"=w547) -> ("error out"=w544:errorcluster, "Data Haso (dup)"=w545:T4)  [unwired: 3 in]
                              n174 = call "DataHaso phase.vi"("error in (no error)"=w544, "Data Haso"=w545) -> ("error out"=w542:errorcluster, "Phase (µm)"=w543:i32, "Data Haso (dup)"=w529:T4)  [unwired: 3 in]
                              n175 = call "Formatter Intensity Graph.vi"("error in (no error)"=w542, "Intensity Graph"=w530, "Surface with pupil"=w543) -> ("error out"=w540:errorcluster, "Surface with pupil (dup)"=w541:i32)  [unwired: 2 in, 1 out]
                              n176 = call "Surface with pupil get stats.vi"("error in (no error)"=w540, "Surface Avec Pupille"=w541) -> ("error out"=w561:errorcluster, "PV"=w526:sgl, "RMS"=w527:dbl)  [unwired: 2 in, 1 out]
                              "RMS" <- w527
                              "PV" <- w526
                              n177 = Merge Errors(w561, w552) -> (w560:errorcluster)
                              n178 = Bundle By Name(cluster=T6 {"Target for tilt"=0, "Target for focus"=0, "Target for all other aberrations"=0} ("References"), "Target for tilt"=w510, "Target for focus"=w510) -> (w564:T6)
                              n179 = call "DataHaso ctor copie.vi"("error in (no error)"=w560, "DataHaso"=w529) -> ("error out"=w563:errorcluster, "new DataHaso"=w562:T4, "DataHaso (dup)"=w528:T4)  [unwired: 3 in]
                              n180 = call "Casao Compute target.vi"("error in (no error)"=w563, "Targets"=w564, "DataHaso"=w562, "Casao"=w553) -> ("error out"=w558:errorcluster, "DataHaso (dup)"=w532:T4, "Casao (dup)"=w559:T10)  [unwired: 1 out]
                              n181 = Bundle By Name(cluster=T5 {"Measurement"=0, "Target"=0, "Manual target"=0} ("Slopes"), "Measurement"=w528, "Target"=w532) -> (w557:T5)
                              n182 = call "Casao get correction commands.vi"("Casao"=w559, "Slopes"=w557, "error in (no error)"=w558) -> ("Casao (dup)"=w531:T10, "Commands"=w524:sgl[], "error out"=w504:errorcluster)  [unwired: 2 in, 2 out]
                              n183 = case shown="True" w507 {
                                tunnel: w504 -> [_ w571]
                                tunnel: w524 -> [_ w570]
                                tunnel: w511 -> [_ w569]
                                frame False {
                                }
                                frame True {
                                n184 = call "PhaseModul apply command.vi"("error in (no error)"=w571, "Commands in"=w570, "Mirror"=w569) -> ()  [unwired: 2 in, 3 out]
                                }
                              }
                            }
                            frame #4 {
                              n185 = call "DataHaso dtor.vi"("Data Haso"=w580) -> ()  [unwired: 6 in, 1 out]
                              n186 = case shown="Error" w574 {
                                tunnel: w573 -> [w581 _]
                                tunnel: [w581 w582] -> w572
                                frame No Error {
                                }
                                frame Error {
                                n187 = Initialize Array(0.0 ("element"), 52 ("dimension size")) -> (w582:dbl[])
                                }
                              }
                            }
                          }
                        }
                      }
                      frame #4 {
                        n188 = call "DataHaso dtor.vi"("Data Haso"=w590) -> ()  [unwired: 6 in, 1 out]
                        n189 = local read "Slice now"() -> (w595:dbl)
                        n190 = Cluster To Array(cluster=w601) -> (array=w600:sgl[])
                        n191 = Build Array (concatenate)(w602, w603, w600, w592) -> (w608:dbl[])
                        n192 = Number To Decimal String(number=w595) -> (decimal integer string=w605:string)  [unwired: 1 in]
                        n193 = Number To Decimal String(number=w595) -> (decimal integer string=w597:string)  [unwired: 1 in]
                        n194 = call "AO single value.vi"("data"=0.0, "physical channels"=tag "Dev1/ao4") -> ()  [unwired: 1 in, 1 out]
                        n195 = call "AO single value.vi"("data"=-5.0, "physical channels"=tag "Dev1/ao5") -> ()  [unwired: 1 in, 1 out]
                        n196 = local read "output path"() -> (w589:path)
                        n197 = Concatenate Strings("afterC_slice", w605, ".dat") -> (w588:string)
                        n198 = Concatenate Strings("command", w597, ".dat") -> (w586:string)
                        n199 = Build Path(base path=w589, name or relative path=w588) -> (appended path=w587:path)
                        n200 = Build Path(base path=w589, name or relative path=w586) -> (appended path=w585:path)
                        n201 = call-poly <vilib>:"Write To Spreadsheet File.vi"("transpose? (no:F)"=TRUE, "format (%.3f)"="%.6f", "1D data"=w608, "file path (dialog if empty)"=w587) -> ()  [unwired: 4 in, 1 out]
                        n202 = call-poly <vilib>:"Write To Spreadsheet File.vi"("transpose? (no:F)"=TRUE, "format (%.3f)"="%.6f", "1D data"=w591, "file path (dialog if empty)"=w585) -> ()  [unwired: 4 in, 1 out]
                      }
                      frame #5 {
                        n203 = local read "Average Frame #"() -> (w615:dbl)
                        n204 = for {
                          N: w615 -> [_]
                          n205 = local read "stop"() -> (w616:bool)
                          n206 = Not(x=w616) -> (.not. x?=w617:bool)
                          n207 = case shown="True" w617 {
                            frame False {
                            }
                            frame True {
                              n208 = flat-sequence {
                                frame #0 {
                                n209 = local read "Laser Power%(0-100)"() -> (w619:dbl)
                                n210 = local read "ImExp Time (s)"() -> (w620:dbl)
                                n211 = local read "Scale factor"() -> (w618:dbl)
                                n212 = call "waveform gen_scale factor.vi"("Scale factor"=w618, "Boolean"=TRUE, "Exposure Time (s)"=w620, "Laser Power%(0-100)"=w619) -> ("waveform"=w622:waveform(dbl)[])
                                n213 = Index Array(array=w622, index=4) -> (element=w630:waveform(dbl))
                                n214 = call "AO triggle.vi"("physical channels"=tag "Dev1/ao0:4", "data"=w622, "waveform"=w630, "trig source"=tag "/Dev1/PFI1") -> ("task out"=w627:refnum<k21>, "error out"=w624:errorcluster)  [unwired: 1 in]
                                n215 = call "DO single value.vi"("error in"=w624, "data"=TRUE, "lines"=tag "Dev1/port0/line0") -> ("error out"=w623:errorcluster)
                                n216 = while {
                                tunnel: [w638] -> w633
                                tunnel: [w637] -> w632
                                tunnel: w627 -> [w635]
                                tunnel: w623 -> [w634]
                                stop <- w636 stop-if-true
                                n217 = call <vilib>:"DAQmx Is Task Done.vi"("task/channels in"=w635, "error in"=w634) -> ("task out"=w638:refnum<k21>, "task done?"=w636:bool, "error out"=w637:errorcluster)  [unwired: 11 in]
                                }
                                n218 = call <vilib>:"DAQmx Clear Task.vi"("task in"=w633, "error in"=w632) -> ()  [unwired: 13 in, 1 out]
                                }
                                frame #1 {
                                n219 = call "AO single value.vi"("data"=0.0, "physical channels"=tag "Dev1/ao4") -> ()  [unwired: 1 in, 1 out]
                                n220 = call "DO single value.vi"("data"=FALSE, "lines"=tag "Dev1/port0/line0") -> ()  [unwired: 1 in, 1 out]
                                }
                              }
                            }
                          }
                        }
                      }
                      frame #6 {
                        n221 = local read "Step size(um)"() -> (w649:dbl)
                        n222 = Multiply(x=w649, y=10.0) -> (x*y=w647:dbl)
                        n223 = Number To Decimal String(number=w647) -> (decimal integer string=w644:string)  [unwired: 1 in]
                        n224 = Concatenate Strings("movrel z=", w644) -> (w645:string)
                        n225 = call "WriteCmd.vi"("Command"=w645, "VISA resource name"=refnum<visa-resource-name> "COM1") -> ()  [unwired: 1 in, 1 out]
                      }
                      frame #7 {
                        n226 = Wait (ms)(milliseconds to wait=u32 50) -> ()  [unwired: 1 out]
                      }
                    }
                  }
                }
                n227 = call "AO single value.vi"("data"=0.0, "physical channels"=tag "Dev1/ao4") -> ()  [unwired: 1 in, 1 out]
              }
            }
            frame #2 {
              n228 = call "Casao dtor.vi"("Casao"=w651) -> ()  [unwired: 6 in, 1 out]
            }
          }
        }
      }
    }
    frame #2 {
      n229 = local read "Step size(um)"() -> (w659:dbl)
      n230 = local read "Slices #"() -> (w652:dbl)
      n231 = Multiply(x=w659, y=-10.0) -> (x*y=w660:dbl)
      n232 = Multiply(x=w660, y=w652) -> (x*y=w658:dbl)
      n233 = Number To Decimal String(number=w658) -> (decimal integer string=w654:string)  [unwired: 1 in]
      n234 = Concatenate Strings("movrel z=", w654) -> (w655:string)
      n235 = call "AO single value.vi"("data"=0.0, "physical channels"=tag "Dev1/ao4") -> ()  [unwired: 1 in, 1 out]
      n236 = call "WriteCmd.vi"("Command"=w655, "VISA resource name"=refnum<visa-resource-name> "COM1") -> ()  [unwired: 1 in, 1 out]
      n237 = call "DO single value.vi"("data"=FALSE, "lines"=tag "Dev1/port0/line1") -> ()  [unwired: 1 in, 1 out]
      n238 = call "DO single value.vi"("data"=FALSE, "lines"=tag "Dev1/port0/line0") -> ()  [unwired: 1 in, 1 out]
    }
  }
